vi "Dashboard Main.vi"() -> ()   [LabVIEW 2016]
uses:
  <vilib>/Utility/miscctls.llb/LVRowAndColumnTypeDef.ctl
  <vilib>/event_ctls.llb/eventvkey.ctl
  <vilib>/Rock Robotics/Network Tables/NT Read Numeric Array.vi
  <vilib>/Rock Robotics/WPI/Dashboard/WPI_DashboardLogging Global.vi
panel:
  in  "rect":T1
  in  "Camera Settings Right":T2={"Frame Rate"=30, "Compression"=30, "Size"=1, "DB Camera Config"=FALSE} {"Frame Rate" scale=1.0..30.0; "Compression" scale=100.0..-1.0; "Size" items=["640x480", "320x240", "160x120"]}
  in  "Camera Name Right":string(combo)="No Camera Selection"
  out "Camera Info":cluster{"Mbps LED":bool, "Mbps":dbl, "fps":dbl} {"fps" format="%#.1g"; "Mbps" format="%#.1g"}
  in  "Camera Settings":T2={"Frame Rate"=30, "Compression"=30, "Size"=1, "DB Camera Config"=FALSE} {"Frame Rate" scale=1.0..30.0; "Compression" scale=100.0..-1.0; "Size" items=["640x480", "320x240", "160x120"]}
  in  "TCP":refnum<k5>
  in  "Rec Mode":enum32{"Stop", "Record", "Playback"}(radio)
  out "Robot IP":string
  out "Image Message":string="Timeout in Camera Communications"
  in  "Dashboard Tab":T3(tab)
  in  "Select Auto":string(combo)="Select Autonomous ..."
  out "NT Connection":bool
  out "MotorChart R":cluster{"Numeric":dbl, "Numeric":dbl}(graph)
  out "MotorChart L":cluster{"Numeric":dbl, "Numeric":dbl}(graph)
  out "MotorSliders R":cluster{"MotorSlide1":dbl, "MotorSlide2":dbl} {"MotorSlide2" scale=-1.0..1.0 scale format="%#_2e"; "MotorSlide1" scale=-1.0..1.0 scale format="%#_2e"}
  out "MotorSliders L":cluster{"MotorSlide1":dbl, "MotorSlide2":dbl} {"MotorSlide2" scale=-1.0..1.0 scale format="%#_2e"; "MotorSlide1" scale=-1.0..1.0 scale format="%#_2e"}
  out "Gyro":dbl(knob) scale=0.0..360.0
  out "JS1 Z":dbl(slide) scale=-1.0..1.0 scale format="%#_2e"
  out "JS1 Graph":cluster{"X":dbl, "Y":dbl}[](graph)
  out "JS1 Buttons":T4
  out "JS2 Z":dbl(slide) scale=-1.0..1.0 scale format="%#_2e"
  out "JS2 Graph":cluster{"X":dbl, "Y":dbl}[](graph)
  out "JS2 Buttons":T4
  out "Mode":T5(ring)=enum."Auto Disabled"
  out "Camera Image Right":T6(plugin-control)
  in  "DB/String 9":string
  in  "DB/String 8":string
  in  "DB/String 7":string
  in  "DB/String 6":string
  in  "DB/String 5":string
  in  "DB/String 4":string
  in  "DB/String 3":string
  in  "DB/String 2":string
  in  "DB/String 1":string
  in  "DB/String 0":string
  in  "DB/Slider 0":dbl(slide) scale=0.0..5.0
  in  "DB/Slider 1":dbl(slide) scale=0.0..5.0
  in  "DB/Slider 2":dbl(slide) scale=0.0..5.0
  in  "DB/Slider 3":dbl(slide) scale=0.0..5.0
  out "DB/LED 3":bool
  out "DB/LED 2":bool
  out "DB/LED 1":bool
  out "DB/LED 0":bool
  in  "DB/Button 3":bool
  in  "DB/Button 2":bool
  in  "DB/Button 1":bool
  in  "DB/Button 0":bool caption="New Name"
  in  "Test Slider":dbl(slide) scale=0.0..100.0 scale format="%#_3g"
  in  "On/Off":bool caption="Solenoid"
  in  "Test Name":u16(ring) items=["Select the test to run..."]
  in  "Test Tree":string(tree)
  in  "Motor":cluster{"Value":dbl, "Enable":bool} {"Value" scale=-1.0..1.0 scale format="%#_3g"}
  out "Progress":T7 {"Test Progress" scale=0.0..100.0}
  in  "Rev/Fwd":cluster{"Forward":bool, "Reverse":bool}
  in  "Test Ring":u16(ring) items=["Monochrome", "Color"]
  out "Cmd Status":string
  in  "Execute Command":bool
  in  "Command Params":string[][](table)
  in  "Command Selection":i32(listbox)
  in  "CheckList":i32(listbox)
  out "Tree":string(tree)
  out "Camera Image":T6(plugin-control)
  out "Background":bool
  in  "Camera Name":string(combo)="No Camera Selection"
  # "HW"
  # "HW"
  # "Joysticks"
  # "Drive Motors"
  # "Front"
  # "Right"
  # "Left"
  # "Back"
  # "This tab is a great place for autonomous settings and robot-specific values.\nPlace controls and indicators inside this tab and match name to\nDashboard Variables on robot. You can also delete this comment."
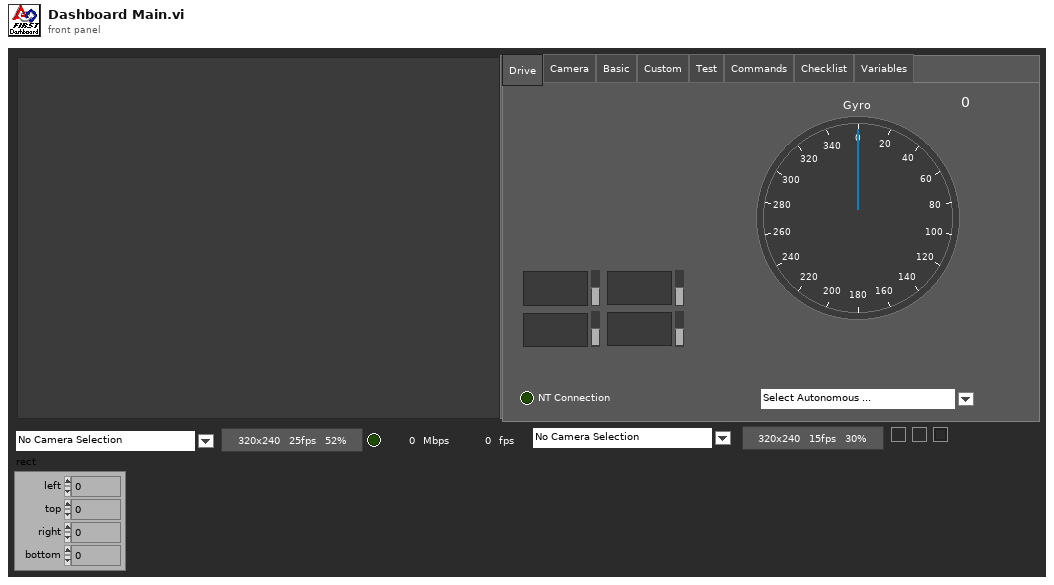
[diagram p1: front panel]
types:
  T1 = cluster{"left":i16, "top":i16, "right":i16, "bottom":i16}
  T2 = cluster{"Frame Rate":i32, "Compression":i32, "Size":u16, "DB Camera Config":bool}
  T3 = enum32{"Drive", "Camera", "Basic", "Custom", "Test", "Commands", "Checklist", "Variables"}
  T4 = cluster{bool, bool, bool, bool, bool, bool, bool, bool, bool, bool, bool, bool}
  T5 = enum8{"Tele-Op Disabled", "Tele-Op Enabled", "Auto Disabled", "Auto Enabled", "Test Disabled", "Test Enabled", "Disconnected", "No Code", "E-Stop"}
  T6 = typedef "IMAQ Image.ctl" = refnum<image>
  T7 = cluster{"Test Progress":u8, "Test Progress Text":string}
  T8 = typedef "Image Type" = u32
  T9 = cluster{"IDs":cluster{"RPC field ID":u16, "Unique ID":u16}, "String":string}
  T10 = enum32{"Drive", "Basic", "Custom", "Test", "Checklist", "Variables"}
  T11 = cluster{"Error Strings":string, "Disable Counts":cluster{u16, u16}, "Rail Faults":cluster{u16, u16, u16}, "Robot IP":string, "DB Mode":u8, "Event Info":cluster{"Name":string, "Type":u8, "Number":u16, "Replay":u8}}
  T12 = cluster{"Storage":cluster{"Disk Free":u64, "RAM Block":u32, "RAM free":u32}, "CPU Utilization":cluster{"CPU % ISR":sgl, "CPU % Time Crit":sgl, "CPU % Timed Str":sgl, "CPU % High":sgl, "CPU % Above":sgl, "CPU % Normal":sgl, "CPU % Low":sgl}, "CAN":cluster{"% Bus Utilization":sgl, "Bus Off Cnt":u32, "TX_FIFO Full Cnt":u32, "Receive Error Cnt":u8, "Transmit Error Cnt":u8}, "HID":cluster{"HID Outputs":u32, "Rumble Low":u16, "Rumble High":u16}[]}
  T13 = cluster{"Status bits":cluster{"Test Mode":bool, "Autonomous":bool, "Enabled":bool, "Code Start":bool, "Brownout":bool, "Reserved 2":bool, "Reserved 3":bool, "E-Stop":bool}, "Code Trace":cluster{"Disabled":bool, "TeleOp":bool, "Auto":bool, "Test":bool}, "Controller Type":enum16{"unknown", "cRIO", "roboRio"}, "Code?":enum16{"unknown", "noCode", "code"}, "Battery V":dbl}
  T14 = cluster{"Control Bits":cluster{"TestMode":bool, "Autonomous":bool, "Enabled":bool, "FMS Present":bool, bool, bool, bool, "E-Stop":bool}, "Team Station ":u8, "Countdown":sgl, "Joystick Values":cluster{"Axes":dbl[], "Buttons":bool[], "POVs":i16[]}[]}
  T15 = cluster{"Axes":dbl[], "Buttons":bool[], "POVs":i16[]}[]
  T16 = cluster{"Axes":dbl[], "Buttons":bool[], "POVs":i16[]}
  T17 = cluster{"Buttons[0]":bool, "Buttons[1]":bool, "Buttons[2]":bool, "Buttons[3]":bool, "Buttons[4]":bool, "Buttons[5]":bool, "Buttons[6]":bool, "Buttons[7]":bool, "Buttons[8]":bool, "Buttons[9]":bool, "Buttons[10]":bool, "Buttons[11]":bool}
  T18 = cluster{"Camera Image":refnum<vi>, "Dashboard Tab":refnum<vi>, "Background":refnum<vi>, "Rec Mode":refnum<vi>, "Test Slider":refnum<vi>, "On/Off ":refnum<vi>, "Test Ring":refnum<vi>, "Rev/Fwd":refnum<vi>, "Test Name":refnum<vi>, "Motor":refnum<vi>, "Progress":refnum<vi>, "CheckList":refnum<vi>, "Tree":refnum<vi>, "Test Tree":refnum<vi>, "Command Params":refnum<vi>, "Command Selection":refnum<vi>, "Execute Command":refnum<vi>, "Cmd Status":refnum<vi>, "Camera Settings":refnum<vi>, "Camera Name":refnum<vi>, "Camera Info":refnum<vi>, "Camera Settings Right":refnum<vi>, "Camera Name Right":refnum<vi>, "Camera Image Right":refnum<vi>}
  T19 = cluster{"Operation":enum16{"Update", "Clear"}, "Color Box":u32}[]
  T20 = typedef "eventvkey.ctl" = enum16{"ASCII", "Enter", "Return", "Shift", "Ctrl", "Alt", "Cmd", "Opt", "Caps", "NumLock", "Clear", "Break", "Up", "Down", "Left", "Right", "Insert", "Delete", "Home", "End", "PageUp", "PageDown", "Escape", "Help", "Pause", "ScrollLock", "F1", "F2", "F3", "F4", "F5", "F6", "F7", "F8", "F9", "F10", "F11", "F12", "F13", "F14", "F15", "F16", "F17", "F18", "F19", "F20", "F21", "F22", "F23", "F24", "Play", "VolumeUp", "VolumeDown", "Mute", "Two Byte Char"}
  T21 = cluster{"Image Size":bool, "Image Type":bool, "Pixel Value":bool, "ROI Information":bool, "Zoom Factor":bool}
  T22 = cluster{"Operation":enum16{"Update", "Clear"}, "Color Box":u32}
  T23 = typedef "LVRowAndColumnTypeDef.ctl" = cluster{"Row":i32, "Column":i32}
  T24 = cluster{"Shift":bool, "Ctrl":bool, "Alt":bool, "Cmd":bool, "Opt":bool}
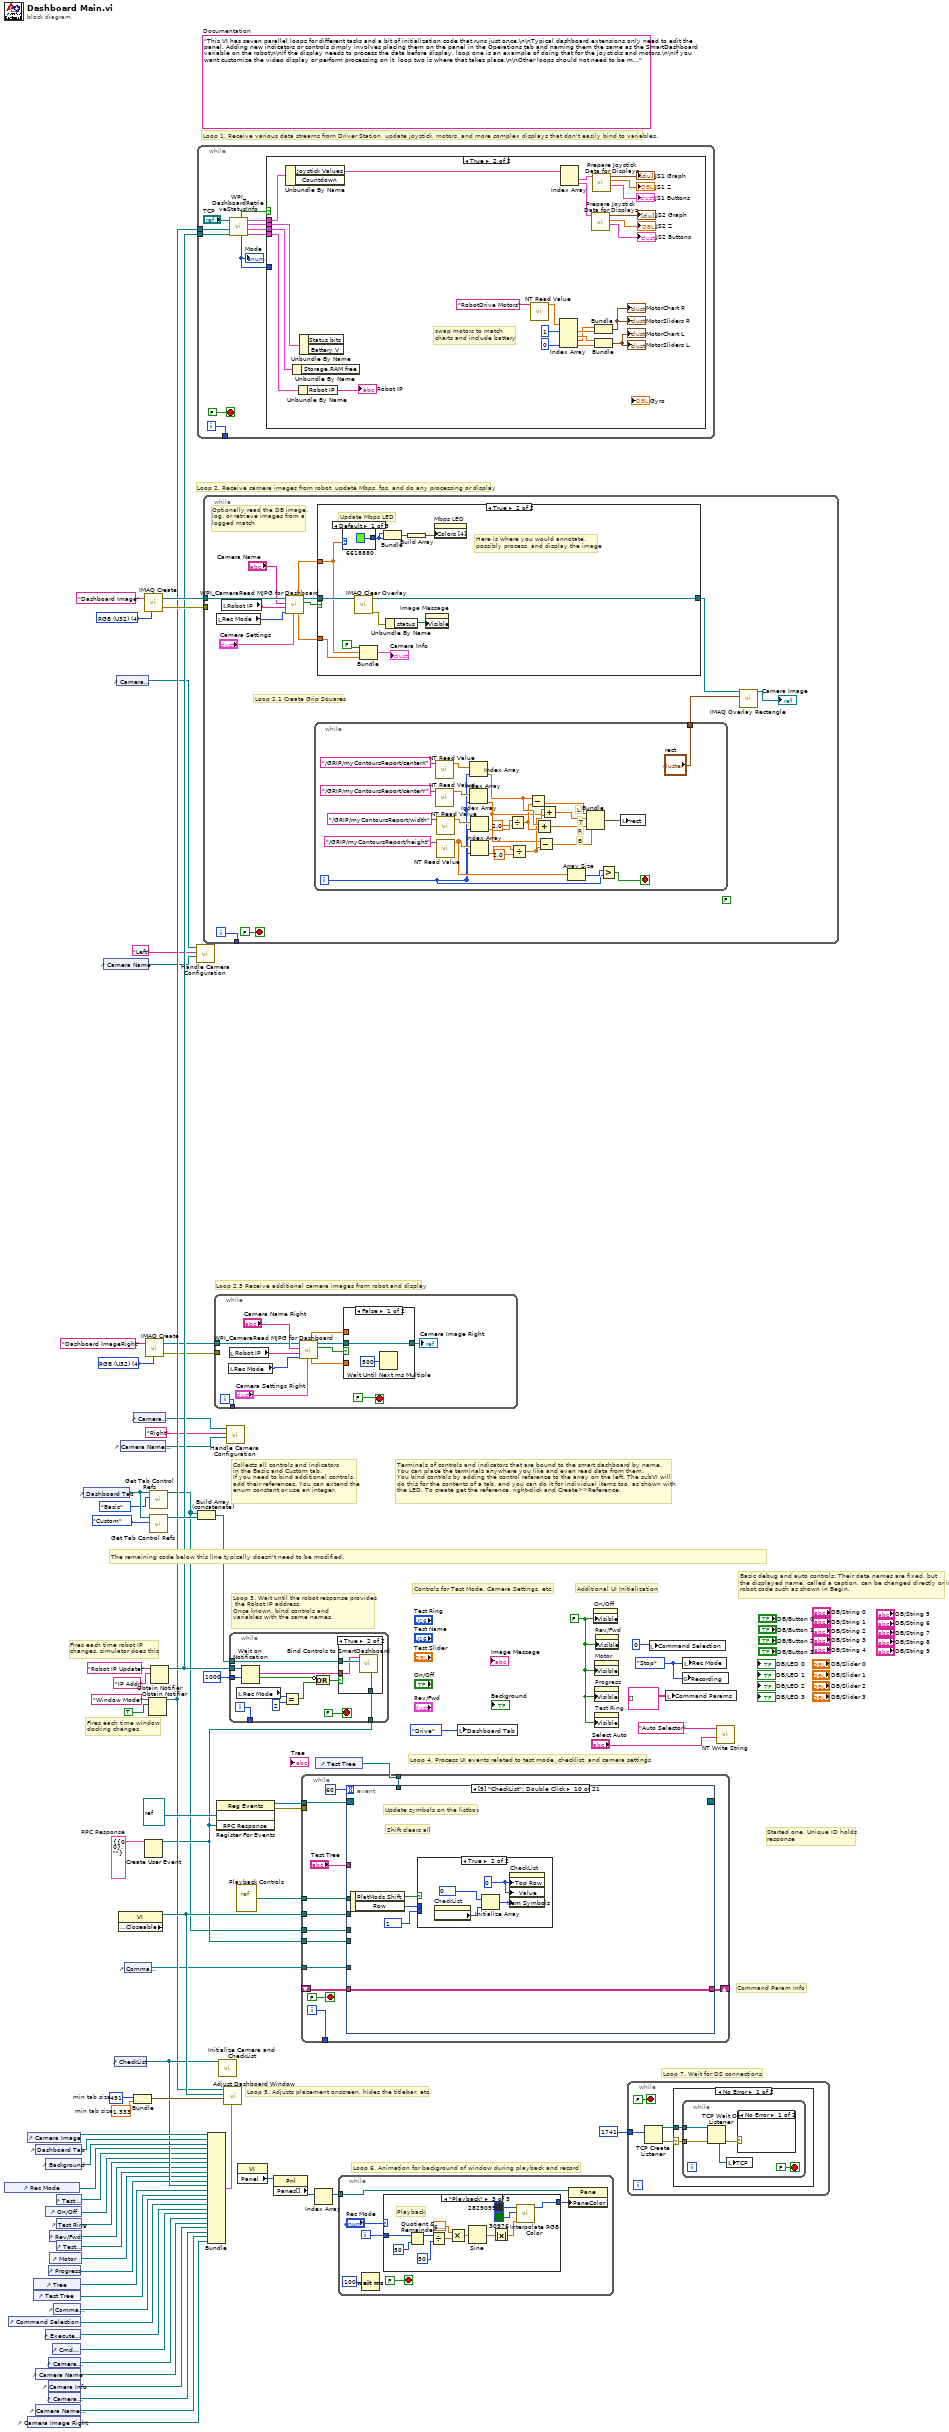
[diagram p0: block diagram]
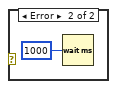
[diagram p3: hidden frame]
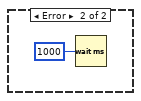
[diagram p4: hidden frame]
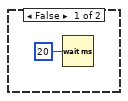
[diagram p5: hidden frame]
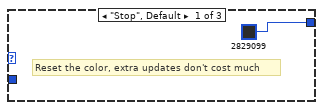
[diagram p6: hidden frame]
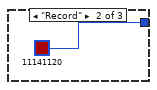
[diagram p7: hidden frame]
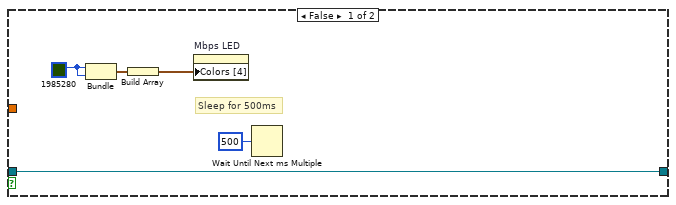
[diagram p9: hidden frame]
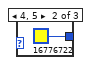
[diagram p10: hidden frame]
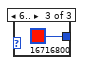
[diagram p11: hidden frame]
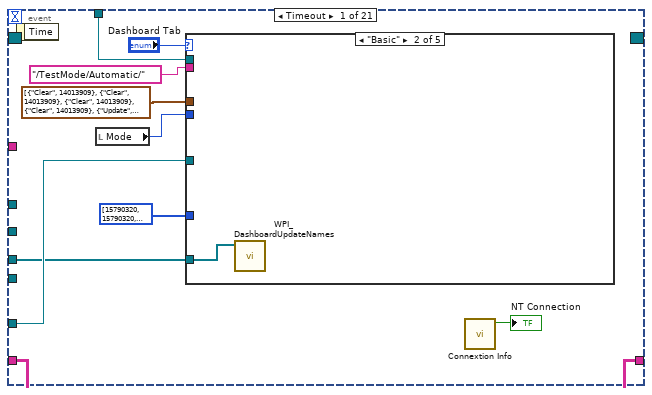
[diagram p12: hidden frame]
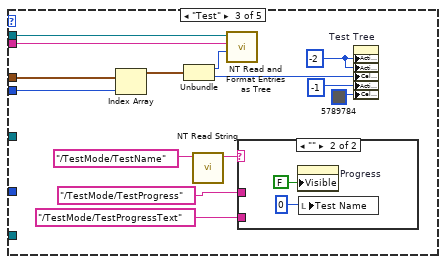
[diagram p14: hidden frame]
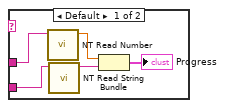
[diagram p15: hidden frame]
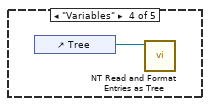
[diagram p16: hidden frame]
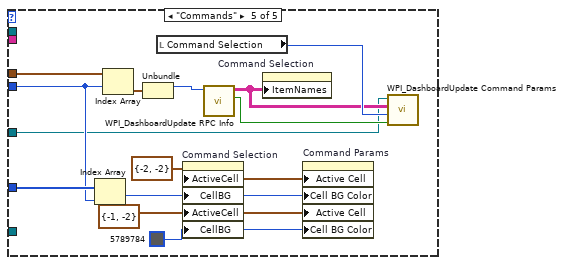
[diagram p17: hidden frame]
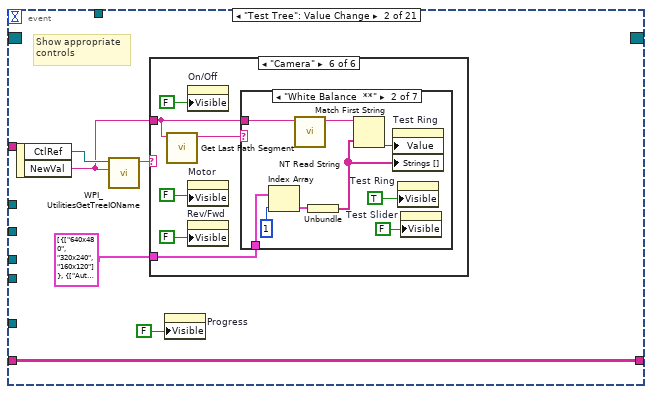
[diagram p18: hidden frame]
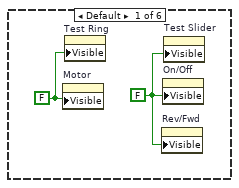
[diagram p19: hidden frame]
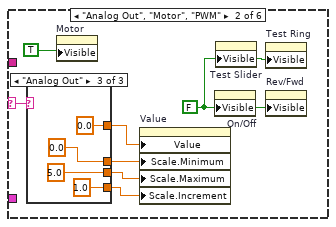
[diagram p20: hidden frame]
diagram:
  w10 = T8 4 items=["Grayscale (U8)", "Grayscale (I16)", "Grayscale (SGL)", "Complex (CSG)", "RGB (U32)", "HSL (U32)", "RGB (U64)"] ("Image Type")
  w26 = T9 {"IDs"={"RPC field ID"=0, "Unique ID"=0}, "String"=""}  # RPC Response
  w51 = 491  # min tab size
  w50 = 1.333  # min tab size
  w58 = enum32{"Stop", "Record", "Playback"}."Stop" ("Rec Mode")
  w33 = FALSE ("Visible")
  (unwired) "This VI has seven parallel loops for different tasks and a bit of initialization code that runs just once.\n\nTypical dashboard extensions only need to edit the panel. Adding new indicators or controls simply involves placing them on the panel in the Operations tab and naming them the same as the SmartDashboard variable on the robot\n\nIf the display needs to process the data before display, loop one is an example of doing that for the joysticks and motors.\n\nIf you want customize the video display or perform processing on it, loop two is where that takes place.\n\nOther loops should not need to be modified. They are pretty standard, and document the task they perform."  # Documentation
  w75 = T8 4 items=["Grayscale (U8)", "Grayscale (I16)", "Grayscale (SGL)", "Complex (CSG)", "RGB (U32)", "HSL (U32)", "RGB (U64)"] ("Image Type")
  # "Loop 2.5 Receive additional camera images from robot and display"
  # "Command Param Info"
  # "Started one, Unique ID holds\nresponse"
  # "Loop 7. Wait for DS connections"
  # "Basic debug and auto controls: Their data names are fixed, but\nthe displayed name, called a caption, can be changed directly or in\nrobot code such as shown in Begin."
  # "Controls for Test Mode, Camera Settings, etc."
  # "Additional UI Initialization"
  # "Loop 6. Animation for background of window during playback and record"
  # "Fires each time robot IP\nchanges, simulator does this"
  # "Fires each time window\ndocking changes."
  # "Collects all controls and indicators\nin the Basic and Custom tab.\nIf you need to bind additional controls,\nadd their references. You can extend the\nenum constant or use an integer."
  # "The remaining code below this line typically doesn't need to be modified."
  # "Loop 4. Process UI events related to test mode, checklist, and camera settings"
  # "Terminals of controls and indicators that are bound to the smart dashboard by name.\nYou can place the terminals anywhere you like and even read data from them.\nYou bind controls by adding the control reference to the array on the left. The subVI will\ndo this for the contents of a tab, and you can do it for individual items too, as shown with\nthe LED. To create get the reference, right-click and Create>>Reference."
  # "Loop 3. Wait until the robot response provides\n the Robot IP address.\nOnce known, bind controls and\nvariables with the same names."
  # "Loop 5. Adjusts placement onscreen, hides the titlebar, etc."
  # "Loop 1. Receive various data streams from Driver Station, update joystick, motors, and more complex displays that don't easily bind to variables."
  # "Loop 2. Receive camera images from robot, update Mbps, fps, and do any processing or display"
  n1 = control-ref of="Rec Mode"() -> (w39:refnum<vi>)
  n2 = control-ref of="Command Selection"() -> (w25:refnum<vi>)
  n3 = control-ref of="Camera Image Right"() -> (w1:refnum<vi>)
  n4 = control-ref of="Camera Image"() -> (w53:refnum<vi>)
  n5 = control-ref of="Tree"() -> (w43:refnum<vi>)
  n6 = control-ref of="Test Tree"() -> (w42:refnum<vi>)
  n7 = control-ref of="Dashboard Tab"() -> (w52:refnum<vi>)
  n8 = control-ref of="Camera Name"() -> (w16:refnum<vi>)
  n9 = control-ref of="Camera Name Right"() -> (w2:refnum<vi>)
  n10 = control-ref of="Execute Command"() -> (w27:refnum<vi>)
  n11 = control-ref of="Background"() -> (w48:refnum<vi>)
  n12 = control-ref of="On/Off"() -> (w37:refnum<vi>)
  n13 = control-ref of="Progress"() -> (w34:refnum<vi>)
  n14 = control-ref of="Camera Settings"() -> (w17:refnum<vi>)
  n15 = control-ref of="Camera Info"() -> (w15:refnum<vi>)
  n16 = control-ref of="Camera Settings Right"() -> (w3:refnum<vi>)
  n17 = control-ref of="Rev/Fwd"() -> (w35:refnum<vi>)
  n18 = control-ref of="Motor"() -> (w40:refnum<vi>)
  n19 = control-ref of="Cmd Status"() -> (w21:refnum<vi>)
  n20 = control-ref of="Command Params"() -> (w28:refnum<vi>)
  n21 = control-ref of="Test Slider"() -> (w38:refnum<vi>)
  n22 = control-ref of="Test Ring"() -> (w36:refnum<vi>)
  n23 = control-ref of="Test Name"() -> (w41:refnum<vi>)
  n24 = control-ref of="Dashboard Tab"() -> (w56:refnum<vi>)
  n25 = control-ref of="Camera Name"() -> (w18:refnum<vi>)
  n26 = control-ref of="CheckList"() -> (w44:refnum<vi>)
  n27 = control-ref of="Camera Settings"() -> (w19:refnum<vi>)
  n28 = property class="VI" props=["Front Panel.Closeable"]() -> (reference out=w57:refnum<vi>)  [unwired: 2 in, 2 out]
  n29 = control-ref of="Camera Name Right"() -> (w6:refnum<vi>)
  n30 = control-ref of="Command Params"() -> (w20:refnum<vi>)
  n31 = control-ref of="Camera Settings Right"() -> (w7:refnum<vi>)
  n32 = Bundle("min tab size"=w51, "min tab size"=w50) -> (w49:cluster{"min tab size":i32, "min tab size":dbl})  [unwired: 1 in]
  n33 = call "IMAQ Create"("Image Name"="Dashboard Image", "Image Type"=w75) -> ("New Image"=w73:T6, "error out"=w72:errorcluster)  [unwired: 2 in, 1 out]
  n34 = Create User Event(user event datatype=w26) -> (user event=w22:refnum<user-event>)  [unwired: 1 in, 1 out]
  n35 = call "IMAQ Create"("Image Name"="Dashboard ImageRight", "Image Type"=w10) -> ("New Image"=w9:T6, "error out"=w8:errorcluster)  [unwired: 2 in, 1 out]
  n36 = Obtain Notifier(name (unnamed)="Window Mode", notification data type=TRUE) -> (notifier out=w31:refnum<notifier>)  [unwired: 2 in, 2 out]
  n37 = call <vilib>:"Get Tab Control Refs.vi"("Page Index"=T10."Basic" ("Dashboard Tab"), "TabControl in"=w56) -> ("ControlsOnPage"=w14:refnum<vi>[])  [unwired: 9 in]
  n38 = call <vilib>:"Get Tab Control Refs.vi"("Page Index"=T10."Custom" ("Dashboard Tab"), "TabControl in"=w56) -> ("ControlsOnPage"=w55:refnum<vi>[])  [unwired: 9 in]
  n39 = Obtain Notifier(name (unnamed)="Robot IP Update", notification data type="IP Addr" ("name (unnamed)")) -> (notifier out=w32:refnum<notifier>)  [unwired: 2 in, 2 out]
  n40 = call "Handle Camera Configuration.vi"("CameraNameRef"=w18, "Camera File Name"="Left", "ClusterRef"=w19) -> ()  [unwired: 9 in]
  n41 = Build Array (concatenate)(w14, w55) -> (w54:refnum<vi>[])
  n42 = while {
    tunnel: [w85] -> _
    tunnel: w32 -> [w79]
    tunnel: w31 -> [w76]
    i -> [w85]
    stop <- FALSE stop-if-true
    n43 = call <vilib>:"WPI_DashboardRetrieveStatusInfo.vi"("Binding Refnum"=w79, "Window Mode Notifier"=w76, "TCP Cnx"="TCP") -> ("Power and Errors"=w80:T11, "Robot Metrics"=w83:T12, "Status Info"=w84:T13, "Control Info"=w81:T14, "Robot Mode"=w78:T5, "Process?"=w82:bool)  [unwired: 3 in]
    "Mode" <- w78
    n44 = case shown="True" w82 {
      tunnel: w84 -> [_ w111]
      tunnel: w83 -> [_ w110]
      tunnel: w81 -> [_ w109]
      tunnel: w80 -> [_ w108]
      tunnel: w78 -> [_ _]
      frame False {
        n45 = Wait (ms)(milliseconds to wait=u32 20) -> ()  [unwired: 1 out]
      }
      frame True {
        # "swap motors to match\ncharts and include battery"
        n46 = Unbundle By Name(w109) -> ("Joystick Values"=w99:T15)  [unwired: 1 out]
        n47 = Unbundle By Name(w110) -> ()  [unwired: 1 out]
        n48 = Unbundle By Name(w108) -> ("Robot IP"=→"Robot IP":string)
        n49 = Unbundle By Name(w111) -> ()  [unwired: 2 out]
        n50 = call-poly <vilib>:"NT Read Value.vi"("Name"="RobotDrive Motors") -> ("Numeric Array"=w89:dbl[])  [unwired: 9 in, 1 out]
        n51 = Index Array(array=w89, index #1=1, index #4=0) -> (element #1=w103:dbl, element #2=w104:dbl, element #3=w102:dbl, element #4=w107:dbl)  [unwired: 2 in]
        n52 = Index Array(array=w99) -> (element #1=w98:T16, element #2=w94:T16)  [unwired: 2 in]
        n53 = call "Prepare Joystick Data for Displays.vi"("Joystick Values"=w94) -> ("Buttons"=→"JS2 Buttons":T17, "Z Axis"=→"JS2 Z":dbl, "Cartesian Data"=→"JS2 Graph":cluster{"X axis":dbl, "X axis":dbl}[])  [unwired: 8 in]
        n54 = call "Prepare Joystick Data for Displays.vi"("Joystick Values"=w98) -> ("Buttons"=→"JS1 Buttons":T17, "Z Axis"=→"JS1 Z":dbl, "Cartesian Data"=→"JS1 Graph":cluster{"X axis":dbl, "X axis":dbl}[])  [unwired: 8 in]
        n55 = Bundle("Numeric"=w102, "Numeric"=w103) -> (→"MotorChart R" →"MotorSliders R":cluster{"Numeric":dbl, "Numeric":dbl})  [unwired: 1 in]
        n56 = Bundle("Numeric"=w104, "Numeric"=w107) -> (→"MotorChart L" →"MotorSliders L":cluster{"Numeric":dbl, "Numeric":dbl})  [unwired: 1 in]
      }
    }
  }
  n57 = while {
    tunnel: w73 -> [w123]
    tunnel: w72 -> [_]
    tunnel: [w124] -> _
    i -> [w124]
    stop <- FALSE stop-if-true
    (unwired) FALSE
    # "Loop 2.1 Create Grip Squares"
    # "Optionally read the DB image,\nlog, or retrieve images from a\nlogged match"
    n58 = local read "Rec Mode"() -> (w119:enum32{"Stop", "Record", "Playback"})
    n59 = local read "Robot IP"() -> (w118:string)
    n60 = call <vilib>:"WPI_CameraRead MJPG for Dashboard.vi"("Camera Settings"="Camera Settings", "Rec Mode"=w119, "Robot IP"=w118, "Camera Name"="Camera Name", "Refnum in"=w123) -> ("Active"=w121:bool, "Refnum out"=w122:T6, "FPS"=w120:dbl, "Bandwidth (Mbps)"=w117:dbl)  [unwired: 3 in]
    n61 = while {
      tunnel: ["rect"] -> w114
      i -> [w139]
      stop <- w144 stop-if-true
      # "B"
      # "R"
      # "T"
      # "L"
      n62 = call-poly <vilib>:"NT Read Value.vi"("Name"="/GRIP/myContoursReport/centerX") -> ("Numeric Array"=w143:dbl[])  [unwired: 9 in, 1 out]
      n63 = call-poly <vilib>:"NT Read Value.vi"("Name"="/GRIP/myContoursReport/centerY") -> ("Numeric Array"=w142:dbl[])  [unwired: 9 in, 1 out]
      n64 = call-poly <vilib>:"NT Read Value.vi"("Name"="/GRIP/myContoursReport/height") -> ("Numeric Array"=w140:dbl[])  [unwired: 9 in, 1 out]
      n65 = call-poly <vilib>:"NT Read Value.vi"("Name"="/GRIP/myContoursReport/width") -> ("Numeric Array"=w141:dbl[])  [unwired: 9 in, 1 out]
      n66 = Index Array(array=w143, index=w139) -> (element=w135:dbl)
      n67 = Index Array(array=w142, index=w139) -> (element=w129:dbl)
      n68 = Index Array(array=w141, index=w139) -> (element=w138:dbl)
      n69 = Index Array(array=w140, index=w139) -> (element=w131:dbl)
      n70 = Divide(x=w138, y=2.0) -> (x/y=w134:dbl)
      n71 = Divide(x=w131, y=2.0) -> (x/y=w130:dbl)
      n72 = Subtract(x=w135, y=w134) -> (x-y=w136:dbl)
      n73 = Add(x=w135, y=w134) -> (x+y=w133:dbl)
      n74 = Subtract(x=w129, y=w130) -> (x-y=w128:dbl)
      n75 = Add(x=w129, y=w130) -> (x+y=w127:dbl)
      n76 = Array Size(array=w140) -> (size(s)=w145:i32)
      n77 = Bundle(w136, w127, w133, w128) -> (w146:cluster{dbl, dbl, dbl, dbl})  [unwired: 1 in]
      n78 = Greater?(x=w145, y=w139) -> (0:w144:bool)
      n79 = local write "rect"(w146) -> ()
    }
    n80 = case shown="True" w121 {
      tunnel: w122 -> [w151 w162]
      tunnel: w117 -> [_ w159]
      tunnel: w120 -> [_ w160]
      tunnel: [w151 w156] -> w113
      frame False {
        w153 = u32 1985280 ("Color Box")
        # "Sleep for 500ms"
        n81 = Bundle("Color Box"=w153, "Color Box"=w153) -> (w154:cluster{"Color Box":u32, "Color Box":u32})  [unwired: 1 out]
        n82 = Build Array(w154) -> (w152:cluster{"Color Box":u32, "Color Box":u32}[])
        n83 = property on="Mbps LED" class="Bool (strict)"("Colors [4]"=w152) -> ()  [unwired: 2 in, 2 out]
        n84 = Wait Until Next ms Multiple(millisecond multiple=u32 500) -> ()  [unwired: 1 out]
      }
      frame True {
        # "Here is where you would annotate,\npossibly process, and display the image"
        # "Update Mbps LED"
        n85 = case shown="Default" w159 {
          tunnel: [u32 6618880 ("Color Box") u32 16776722 ("Color Box") u32 16716800 ("Color Box")] -> w163
          frame Default {
          }
          frame 4, 5 {
          }
          frame 6.. {
          }
        }
        n86 = call "IMAQ Clear Overlay"("Image"=w162) -> ("error out"=w165:errorcluster, "Image Out"=w156:T6)  [unwired: 2 in, 7 out]
        n87 = Bundle(FALSE, "Bandwidth (Mbps)"=w159, "FPS"=w160) -> (→"Camera Info":cluster{bool, "Bandwidth (Mbps)":dbl, "FPS":dbl})  [unwired: 1 in]
        n88 = Bundle("Color Box"=w163, "Color Box"=w163) -> (w164:cluster{"Color Box":u32, "Color Box":u32})  [unwired: 1 out]
        n89 = Unbundle By Name(w165) -> ("status"=w166:bool)
        n90 = Build Array(w164) -> (w161:cluster{"Color Box":u32, "Color Box":u32}[])
        n91 = property on="Image Message" class="Str"("Visible"=w166) -> ()  [unwired: 2 in, 2 out]
        n92 = property on="Mbps LED" class="Bool (strict)"("Colors [4]"=w161) -> ()  [unwired: 2 in, 2 out]
      }
    }
    n93 = call "IMAQ Overlay Rectangle"("Rectangle"=w114, "Image"=w113) -> ("Image Out"=→"Camera Image":T6)  [unwired: 8 in, 1 out]
  }
  n94 = Bundle("Camera Image"=w53, "Dashboard Tab"=w52, "Background"=w48, "Rec Mode"=w39, "Test Slider"=w38, "On/Off"=w37, "Test Ring"=w36, "Rev/Fwd"=w35, "Test Name"=w41, "Motor"=w40, "Progress"=w34, "CheckList"=w44, "Tree"=w43, "Test Tree"=w42, "Command Params"=w28, "Command Selection"=w25, "Execute Command"=w27, "Cmd Status"=w21, "Camera Settings"=w17, "Camera Name"=w16, "Camera Info"=w15, "Camera Settings Right"=w3, "Camera Name Right"=w2, "Camera Image Right"=w1) -> (w45:T18)  [unwired: 1 in]
  n95 = while {
    tunnel: w9 -> [w180]
    tunnel: w8 -> [_]
    tunnel: [w174] -> _
    i -> [w174]
    stop <- FALSE stop-if-true
    n96 = local read "Rec Mode"() -> (w178:enum32{"Stop", "Record", "Playback"})
    n97 = local read "Robot IP"() -> (w179:string)
    n98 = call <vilib>:"WPI_CameraRead MJPG for Dashboard.vi"("Camera Settings"="Camera Settings Right", "Rec Mode"=w178, "Robot IP"=w179, "Camera Name"="Camera Name Right", "Refnum in"=w180) -> ("Active"=w173:bool, "Refnum out"=w176:T6, "FPS"=w171:dbl, "Bandwidth (Mbps)"=w172:dbl)  [unwired: 3 in]
    n99 = case shown="False" w173 {
      tunnel: w176 -> [w182 w184]
      tunnel: w172 -> [_ _]
      tunnel: w171 -> [_ _]
      tunnel: [w182 w184] -> w170
      frame False {
        n100 = Wait Until Next ms Multiple(millisecond multiple=u32 500) -> ()  [unwired: 1 out]
      }
      frame True {
      }
    }
    "Camera Image Right" <- w170
  }
  n101 = register-events(refnum<vi> refnum, w22) -> (reference out=w62:refnum<event-registration>, error out=w61:errorcluster)  [unwired: 2 in]
  n102 = call "Initialize Camera and CheckList.vi"("ListBox in"=w44) -> ()  [unwired: 11 in]
  n103 = call "Adjust Dashboard Window.vi"("Sizing Refnums"=w45, "Size Constraints"=w49, "VI"=w57, "WIn Mode"=w31) -> ()  [unwired: 8 in]
  n104 = call "Handle Camera Configuration.vi"("CameraNameRef"=w6, "Camera File Name"="Right", "ClusterRef"=w7) -> ()  [unwired: 9 in]
  n105 = while {
    tunnel: w54 -> [w196]
    tunnel: w32 -> [w194]
    tunnel: [w192] -> _
    tunnel: u32 1000 ("milliseconds to wait") -> [w191]
    tunnel: w22 -> [w185]
    i -> [w192]
    stop <- FALSE stop-if-true
    n106 = local read "Rec Mode"() -> (w187:enum32{"Stop", "Record", "Playback"})
    n107 = Wait on Notification(notifier=w194, timeout in ms (-1)=w191) -> (notification=w193:string, timed out?=w189:bool)  [unwired: 2 in, 2 out]
    n108 = Equal?(x=w187, y=u16 2 ("Rec Mode")) -> (x = y?=w188:bool)
    n109 = Compound Arithmetic op=OR(invert w189, w188) -> (w190:bool)
    n110 = case shown="True" w190 {
      tunnel: w196 -> [_ w199]
      tunnel: w193 -> [_ w198]
      tunnel: w185 -> [_ w197]
      frame False {
      }
      frame True {
        n111 = call <vilib>:"Bind Controls to SmartDashboard.vi"("RPC ref"=w197, "Bound Control Refs"=w199, "Server IP Address"=w198) -> ()  [unwired: 9 in]
      }
    }
  }
  n112 = vi-ref "Playback Controls.vi"() -> (w63:refnum<vi>)
  n113 = property class="VI"() -> ("Panel"=w65:refnum<vi>)  [unwired: 2 in, 2 out]
  n114 = property class="Pnl"(reference=w65) -> ("Panes[]"=w66:refnum<vi>[])  [unwired: 1 in, 2 out]
  n115 = Index Array(array=w66) -> (element=w64:refnum<vi>)  [unwired: 1 in]
  n116 = control-ref of="Test Tree"() -> (w67:refnum<vi>)
  n117 = while {
    tunnel: [w209] -> _
    tunnel: w67 -> [w208]
    tunnel: w63 -> [w207]
    tunnel: w62 -> [w206]
    tunnel: w61 -> [_]
    tunnel: w57 -> [w205]
    tunnel: w22 -> [w204]
    tunnel: w20 -> [w203]
    shift-right: [w202] -> _
    shift-left: _ -> [w201]
    tunnel: w14 -> [w200]
    i -> [w209]
    stop <- FALSE stop-if-true
    n118 = event shown="[9] \"CheckList\": Double Click" {
      selector: w206 -> [_ _ _ _ _ _ _ _ _ _ _ _ _ _ _ _ _ _ _ _ _]
      dyn-events: [_ _ _ _ _ _ _ _ _ _ _ _ _ _ _ _ w465 _ _ _ _] -> _
      timeout: u32 60 ("milliseconds to wait") -> [_ _ _ _ _ _ _ _ _ _ _ _ _ _ _ _ _ _ _ _ _]
      tunnel: w208 -> [w221 _ _ _ _ _ _ _ _ _ _ _ _ _ _ _ _ _ _ _ _]
      tunnel: "Test Tree" -> [_ _ _ _ _ _ _ _ _ _ _ w432 w440 w442 w446 w454 _ _ _ _ _]
      tunnel: w207 -> [_ _ _ _ _ _ _ _ _ _ _ _ _ _ _ _ w467 _ w485 _ _]
      tunnel: w205 -> [_ _ _ _ _ _ _ _ _ _ _ _ _ _ _ _ w463 _ _ _ _]
      tunnel: w204 -> [_ _ _ _ _ _ _ _ _ _ _ _ _ _ _ _ w459 _ _ _ _]
      tunnel: w203 -> [w216 _ _ _ _ _ w383 _ _ _ _ _ _ _ _ _ _ _ _ _ _]
      tunnel: [w215 w260 w362 w367 w376 w380 w381 w390 w400 w407 w419 w431 w438 w441 w445 w453 w458 w480 w482 w486 w497] -> w202
      tunnel: w201 -> [w215 w260 w362 w367 w376 w380 w381 _ _ w407 w419 w431 w438 w441 w445 w453 w458 w480 w482 w486 w497]
      tunnel: w200 -> [w213 _ _ _ _ _ _ _ _ _ _ _ _ _ _ _ _ _ _ _ _]
      event Timeout {
        n119 = event-data() -> ()  [unwired: 1 in, 1 out]
        n120 = local read "Mode"() -> (w218:T5)
        n121 = case shown="\"Basic\"" "Dashboard Tab" {
          tunnel: w221 -> [_ _ w237 _ _]
          tunnel: "/TestMode/Automatic/" ("Name Pattern") -> [_ _ w236 _ _]
          tunnel: T19 [{"Operation"=enum."Clear", "Color Box"=14013909}, {"Operation"=enum."Clear", "Color Box"=14013909}, {"Operation"=enum."Clear", "Color Box"=14013909}, {"Operation"=enum."Clear", "Color Box"=14013909}, {"Operation"=enum."Update", "Color Box"=14013909}, {"Operation"=enum."Update", "Color Box"=16777215}, {"Operation"=enum."Clear", "Color Box"=14013909}, {"Operation"=enum."Clear", "Color Box"=14013909}, {"Operation"=enum."Clear", "Color Box"=14013909}] -> [_ _ w229 _ w253]
          tunnel: w218 -> [_ _ w228 _ w252]
          tunnel: u32[] [15790320, 15790320, 15790320, 15790320, 16777215, 16777215, 15790320, 15790320, 15790320] -> [_ _ _ _ w258]
          tunnel: w216 -> [_ _ _ _ w246]
          tunnel: w213 -> [_ w223 _ _ _]
          frame "Custom", Default {
          }
          frame "Basic" {
            n122 = call <vilib>:"WPI_DashboardUpdateNames.vi"("Controls on Tab"=w223) -> ()  [unwired: 11 in]
          }
          frame "Test" {
            w235 = -2 ("Active Item:Row Number")
            n123 = Index Array(array=w229, index=w228) -> (element=w230:T22)
            n124 = Unbundle(w230) -> ("Operation"=w231:enum16{"Update", "Clear"}, "Color Box"=w232:u32)
            n125 = call <vilib>:"NT Read String.vi"("Name"="/TestMode/TestName") -> ("String"=w226:string)  [unwired: 9 in, 1 out]
            n126 = call <vilib>:"NT Read and Format Entries as Tree.vi"("Operation"=w231, "Name Pattern"=w236, "Tree Refnum"=w237) -> ()  [unwired: 7 in, 2 out]
            n127 = case shown="\"\"" w226 {
              tunnel: "/TestMode/TestProgress" ("Name") -> [w239 _]
              tunnel: "/TestMode/TestProgressText" ("Name") -> [w238 _]
              frame Default {
                n128 = call <vilib>:"NT Read Number.vi"("Name"=w239) -> ("Numeric"=w240:dbl)  [unwired: 9 in, 1 out]
                n129 = call <vilib>:"NT Read String.vi"("Name"=w238) -> ("String"=w241:string)  [unwired: 9 in, 1 out]
                n130 = Bundle("Numeric"=w240, "String"=w241) -> (→"Progress":cluster{"Numeric":dbl, "String":string})  [unwired: 1 in]
              }
              frame "" {
                n131 = property on="Progress" class="Clust (strict)"("Visible"=FALSE) -> ()  [unwired: 2 in, 2 out]
                n132 = local write "Test Name"(u16 0) -> ()
              }
            }
            n133 = property on="Test Tree" class="Tree (strict)"("Active Item Row Number"=w235, "ActiveColNum"=w235, "CellBG"=w232, "Active Item Row Number"=-1 ("Active Item:Row Number"), "CellBG"=u32 5789784 ("Color Box")) -> ()  [unwired: 2 in, 2 out]
          }
          frame "Variables" {
            n134 = control-ref of="Tree"() -> (w245:refnum<vi>)
            n135 = call <vilib>:"NT Read and Format Entries as Tree.vi"("Tree Refnum"=w245) -> ()  [unwired: 9 in, 2 out]
          }
          frame "Commands" {
            w254 = u32 5789784 ("Color Box")
            w255 = T23 {"Row"=-1, "Column"=-2} ("Active Cell:Active Cell")
            w257 = T23 {"Row"=-2, "Column"=-2} ("Active Cell:Active Cell")
            n136 = Index Array(array=w258, index=w252) -> (element=w256:u32)
            n137 = Index Array(array=w253, index=w252) -> (element=w251:T22)
            n138 = Unbundle(w251) -> ("Operation"=w250:enum16{"Update", "Clear"})  [unwired: 1 out]
            n139 = local read "Command Selection"() -> (w249:i32)
            n140 = property on="Command Selection" class="MCListbox (strict)"("ActiveCell"=w257, "CellBG"=w256, "ActiveCell"=w255, "CellBG"=w254) -> ()  [unwired: 2 in, 2 out]
            n141 = call <vilib>:"WPI_DashboardUpdate RPC Info.vi"("Operation"=w250) -> ("update"=w248:bool, "commands"=w247:string[][])  [unwired: 9 in]
            n142 = property on="Command Selection" class="MCListbox (strict)"("ItemNames"=w247) -> ()  [unwired: 2 in, 2 out]
            n143 = property on="Command Params" class="Tbl (strict)"("Active Cell"=w257, "Cell BG Color"=w256, "Active Cell"=w255, "Cell BG Color"=w254) -> ()  [unwired: 2 in, 2 out]
            n144 = call <vilib>:"WPI_DashboardUpdate Command Params.vi"("Update"=w248, "NewVal"=w249, "Commands"=w247, "Param Tbl"=w246) -> ()  [unwired: 7 in, 1 out]
          }
        }
        n145 = call <vilib>:"Connextion Info.vi"() -> ("Connected"=→"NT Connection":bool)  [unwired: 10 in, 1 out]
      }
      event "Test Tree": Value Change {
        # "Show appropriate\ncontrols"
        n146 = event-data() -> ("CtlRef"=w263:refnum<vi>, "NewVal"=w261:string)  [unwired: 1 in]
        n147 = call <vilib>:"WPI_UtilitiesGetTreeIOName.vi"("NewVal"=w261, "TreeControl in"=w263) -> ("I/O Name"=w264:string)  [unwired: 9 in]
        n148 = case shown="\"Camera\"" w264 {
          selector: w264 -> [_ w271 _ w293 w302 _]
          tunnel: w261 -> [_ _ w290 w292 _ w309]
          tunnel: cluster{string[]}[] [{["640x480", "320x240", "160x120"]}, {["Auto", "Fixed indoor", "Fixed outdoor 1", "Fixed outdoor 2", "Fixed fluorescent 1", "Fixed fluorescent 2", "Hold current"]}, {["Auto", "Flicker-free 50 Hz", "Flicker-free 60 Hz", "Hold current"]}, {["None", "Prioritize frame rate", "Prioritize image quality"]}, {["Monochrome", "Color"]}] -> [_ _ _ _ _ w308]
          frame Default {
            w266 = FALSE ("Visible")
            w265 = FALSE ("Visible")
            n149 = property on="Motor" class="Clust (strict)"("Visible"=w265) -> ()  [unwired: 2 in, 2 out]
            n150 = property on="Test Ring" class="Ring (strict)"("Visible"=w265) -> ()  [unwired: 2 in, 2 out]
            n151 = property on="Rev/Fwd" class="Clust (strict)"("Visible"=w266) -> ()  [unwired: 2 in, 2 out]
            n152 = property on="On/Off" class="Bool (strict)"("Visible"=w266) -> ()  [unwired: 2 in, 2 out]
            n153 = property on="Test Slider" class="Slide (strict)"("Visible"=w266) -> ()  [unwired: 2 in, 2 out]
          }
          frame "Analog Out", "Motor", "PWM" {
            w272 = FALSE ("Visible")
            n154 = case shown="\"Analog Out\"" w271 {
              tunnel: [1.0 ("Value") -1.0 ("Value") 0.0 ("Value")] -> w270
              tunnel: [255.0 ("Value") 1.0 ("Value") 5.0 ("Value")] -> w269
              tunnel: [128.0 ("Value") 0.0 ("Value") 0.0 ("Value")] -> w268
              tunnel: [64.0 ("Value") 0.5 ("Value") 1.0 ("Value")] -> w267
              frame "PWM" {
              }
              frame "Motor", Default {
              }
              frame "Analog Out" {
              }
            }
            n155 = property on="Motor" class="Clust (strict)"("Visible"=TRUE) -> ()  [unwired: 2 in, 2 out]
            n156 = property on="Value" class="Slide (strict)"("Value"=w268, "Scale.Minimum"=w270, "Scale.Maximum"=w269, "Scale.Increment"=w267) -> ()  [unwired: 2 in, 2 out]
            n157 = property on="On/Off" class="Bool (strict)"("Visible"=w272) -> ()  [unwired: 2 in, 2 out]
            n158 = property on="Test Slider" class="Slide (strict)"("Visible"=w272) -> ()  [unwired: 2 in, 2 out]
            n159 = property on="Test Ring" class="Ring (strict)"("Visible"=w272) -> ()  [unwired: 2 in, 2 out]
            n160 = property on="Rev/Fwd" class="Clust (strict)"("Visible"=w272) -> ()  [unwired: 2 in, 2 out]
          }
          frame "Servo" {
            w288 = FALSE ("Visible")
            n161 = call <vilib>:"NT Read Number.vi"("Name"=w290) -> ("Numeric"=w289:dbl)  [unwired: 9 in, 1 out]
            n162 = property on="Test Slider" class="Slide (strict)"("Visible"=TRUE, "Scale.Maximum"=170.0 ("Scale.Range:Maximum")) -> ()  [unwired: 2 in, 2 out]
            n163 = local write "Test Slider"(w289) -> ()
            n164 = property on="Motor" class="Clust (strict)"("Visible"=w288) -> ()  [unwired: 2 in, 2 out]
            n165 = property on="Rev/Fwd" class="Clust (strict)"("Visible"=w288) -> ()  [unwired: 2 in, 2 out]
            n166 = property on="On/Off" class="Bool (strict)"("Visible"=w288) -> ()  [unwired: 2 in, 2 out]
            n167 = property on="Test Ring" class="Ring (strict)"("Visible"=w288) -> ()  [unwired: 2 in, 2 out]
          }
          frame "Relay", "Solenoid" {
            w291 = FALSE ("Visible")
            n168 = property on="Motor" class="Clust (strict)"("Visible"=w291) -> ()  [unwired: 2 in, 2 out]
            n169 = property on="Test Slider" class="Slide (strict)"("Visible"=w291) -> ()  [unwired: 2 in, 2 out]
            n170 = Search and Replace String(input string=w292, search string="/Value  **", replace string="/Direction") -> (result string=w298:string)  [unwired: 5 in, 3 out]
            n171 = property on="Test Ring" class="Ring (strict)"("Visible"=w291) -> ()  [unwired: 2 in, 2 out]
            n172 = call <vilib>:"NT Read String.vi"("Name"=w298) -> ("String"=w296:string)  [unwired: 9 in, 1 out]
            n173 = Equal?(x="Both directions", y=w296) -> (x = y?=w294:bool)
            n174 = Not(x=w294) -> (.not. x?=w295:bool)
            n175 = property on="Rev/Fwd" class="Clust (strict)"("Visible"=w294) -> ()  [unwired: 2 in, 2 out]
            n176 = property on="On/Off" class="Bool (strict)"("Visible"=w295, "Caption.Text"=w293) -> ()  [unwired: 2 in, 2 out]
          }
          frame "Compressor", "Digital Out" {
            w301 = FALSE ("Visible")
            # "Get direction and finish"
            n177 = property on="Motor" class="Clust (strict)"("Visible"=w301) -> ()  [unwired: 2 in, 2 out]
            n178 = property on="Test Slider" class="Slide (strict)"("Visible"=w301) -> ()  [unwired: 2 in, 2 out]
            n179 = property on="Test Ring" class="Ring (strict)"("Visible"=w301) -> ()  [unwired: 2 in, 2 out]
            n180 = property on="On/Off" class="Bool (strict)"("Visible"=TRUE, "Caption.Text"=w302) -> ()  [unwired: 2 in, 2 out]
            n181 = property on="Rev/Fwd" class="Clust (strict)"("Visible"=FALSE) -> ()  [unwired: 2 in, 2 out]
          }
          frame "Camera" {
            n182 = call <vilib>:"Get Last Path Segment.vi"("String in"=w309) -> ("String out"=w310:string)  [unwired: 10 in]
            n183 = property on="On/Off" class="Bool (strict)"("Visible"=FALSE) -> ()  [unwired: 2 in, 2 out]
            n184 = property on="Motor" class="Clust (strict)"("Visible"=FALSE) -> ()  [unwired: 2 in, 2 out]
            n185 = property on="Rev/Fwd" class="Clust (strict)"("Visible"=FALSE) -> ()  [unwired: 2 in, 2 out]
            n186 = case shown="\"White Balance  **\"" w310 {
              tunnel: w309 -> [w316 w325 w334 w343 w352 _ w358]
              tunnel: w308 -> [w314 w322 w331 w340 w349 _ _]
              frame "Size  **" {
                n187 = Index Array(array=w314) -> (element=w313:cluster{string[]})  [unwired: 1 in]
                n188 = call <vilib>:"NT Read String.vi"("Name"=w316) -> ("String"=w315:string)  [unwired: 9 in, 1 out]
                n189 = Unbundle(w313) -> (w311:string[])
                n190 = Match First String(2:w311, 3:w315) -> (0:w312:i32)  [unwired: 1 out]
                n191 = property on="Test Ring" class="Ring (strict)"("Value"=w312, "Strings []"=w311) -> ()  [unwired: 2 in, 2 out]
                n192 = property on="Test Ring" class="Ring (strict)"("Visible"=TRUE) -> ()  [unwired: 2 in, 2 out]
                n193 = property on="Test Slider" class="Slide (strict)"("Visible"=FALSE) -> ()  [unwired: 2 in, 2 out]
              }
              frame "White Balance  **" {
                n194 = Index Array(array=w322, index=1) -> (element=w323:cluster{string[]})
                n195 = call <vilib>:"NT Read String.vi"("Name"=w325) -> ("String"=w324:string)  [unwired: 9 in, 1 out]
                n196 = Unbundle(w323) -> (w320:string[])
                n197 = Match First String(2:w320, 3:w324) -> (0:w319:i32)  [unwired: 1 out]
                n198 = property on="Test Ring" class="Ring (strict)"("Value"=w319, "Strings []"=w320) -> ()  [unwired: 2 in, 2 out]
                n199 = property on="Test Ring" class="Ring (strict)"("Visible"=TRUE) -> ()  [unwired: 2 in, 2 out]
                n200 = property on="Test Slider" class="Slide (strict)"("Visible"=FALSE) -> ()  [unwired: 2 in, 2 out]
              }
              frame "Exposure  **" {
                n201 = Index Array(array=w331, index=2) -> (element=w332:cluster{string[]})
                n202 = call <vilib>:"NT Read String.vi"("Name"=w334) -> ("String"=w333:string)  [unwired: 9 in, 1 out]
                n203 = Unbundle(w332) -> (w328:string[])
                n204 = Match First String(2:w328, 3:w333) -> (0:w329:i32)  [unwired: 1 out]
                n205 = property on="Test Ring" class="Ring (strict)"("Value"=w329, "Strings []"=w328) -> ()  [unwired: 2 in, 2 out]
                n206 = property on="Test Ring" class="Ring (strict)"("Visible"=TRUE) -> ()  [unwired: 2 in, 2 out]
                n207 = property on="Test Slider" class="Slide (strict)"("Visible"=FALSE) -> ()  [unwired: 2 in, 2 out]
              }
              frame "Exposure Priority  **" {
                n208 = Index Array(array=w340, index=3) -> (element=w341:cluster{string[]})
                n209 = call <vilib>:"NT Read String.vi"("Name"=w343) -> ("String"=w342:string)  [unwired: 9 in, 1 out]
                n210 = Unbundle(w341) -> (w337:string[])
                n211 = Match First String(2:w337, 3:w342) -> (0:w338:i32)  [unwired: 1 out]
                n212 = property on="Test Ring" class="Ring (strict)"("Value"=w338, "Strings []"=w337) -> ()  [unwired: 2 in, 2 out]
                n213 = property on="Test Ring" class="Ring (strict)"("Visible"=TRUE) -> ()  [unwired: 2 in, 2 out]
                n214 = property on="Test Slider" class="Slide (strict)"("Visible"=FALSE) -> ()  [unwired: 2 in, 2 out]
              }
              frame "Color Enable  **" {
                n215 = Index Array(array=w349, index=4) -> (element=w350:cluster{string[]})
                n216 = call <vilib>:"NT Read String.vi"("Name"=w352) -> ("String"=w351:string)  [unwired: 9 in, 1 out]
                n217 = Unbundle(w350) -> (w346:string[])
                n218 = Match First String(2:w346, 3:w351) -> (0:w347:i32)  [unwired: 1 out]
                n219 = property on="Test Ring" class="Ring (strict)"("Value"=w347, "Strings []"=w346) -> ()  [unwired: 2 in, 2 out]
                n220 = property on="Test Ring" class="Ring (strict)"("Visible"=TRUE) -> ()  [unwired: 2 in, 2 out]
                n221 = property on="Test Slider" class="Slide (strict)"("Visible"=FALSE) -> ()  [unwired: 2 in, 2 out]
              }
              frame Default {
                n222 = property on="Test Ring" class="Ring (strict)"("Visible"=FALSE) -> ()  [unwired: 2 in, 2 out]
                n223 = property on="Test Slider" class="Slide (strict)"("Visible"=FALSE) -> ()  [unwired: 2 in, 2 out]
              }
              frame "Brightness  **", "Color Level  **", "Compression  **", "FPS  **", "Sharpness  **" {
                n224 = call <vilib>:"NT Read Number.vi"("Name"=w358) -> ("Numeric"=w357:dbl)  [unwired: 9 in, 1 out]
                n225 = local write "Test Slider"(w357) -> ()
                n226 = property on="Test Slider" class="Slide (strict)"("Visible"=TRUE, "Scale.Maximum"=100.0 ("Scale.Range:Maximum")) -> ()  [unwired: 2 in, 2 out]
                n227 = property on="Test Ring" class="Ring (strict)"("Visible"=FALSE) -> ()  [unwired: 2 in, 2 out]
              }
            }
          }
        }
        n228 = property on="Progress" class="Clust (strict)"("Visible"=FALSE) -> ()  [unwired: 2 in, 2 out]
      }
      event "Test Name": Mouse Enter {
        # "Populate the ring with the list of tests"
        n229 = event-data() -> ()  [unwired: 1 in, 1 out]
        n230 = call <vilib>:"NT Read String Array.vi"("Name"="/TestMode/TestList") -> ("String Array"=w366:string[])  [unwired: 9 in, 1 out]
        n231 = Build Array (concatenate)("Select the test to run...", w366) -> (w365:string[])
        n232 = property on="Test Name" class="Ring (strict)"("Strings []"=w365) -> ()  [unwired: 2 in, 2 out]
      }
      event "Test Name": Value Change {
        w368 = FALSE ("Visible")
        # "Tell the robot the test name to run"
        n233 = event-data() -> ("NewVal"=w372:u16)  [unwired: 1 in]
        n234 = property on="Test Name" class="Ring (strict)"() -> ("Strings []"=w373:string[])  [unwired: 2 in, 2 out]
        n235 = local write "Progress"(T7 {"Test Progress"=0, "Test Progress Text"=""} ("Progress")) -> ()
        n236 = Index Array(array=w373, index=w372) -> (element=w371:string)
        n237 = call <vilib>:"NT Write String.vi"("String"=w371, "Name"="/TestMode/TestName") -> ()  [unwired: 9 in, 1 out]
        n238 = property on="Progress" class="Clust (strict)"("Visible"=TRUE) -> ()  [unwired: 2 in, 2 out]
        n239 = property on="Motor" class="Clust (strict)"("Visible"=w368) -> ()  [unwired: 2 in, 2 out]
        n240 = property on="Test Slider" class="Slide (strict)"("Visible"=w368) -> ()  [unwired: 2 in, 2 out]
        n241 = property on="On/Off" class="Bool (strict)"("Visible"=w368) -> ()  [unwired: 2 in, 2 out]
        n242 = property on="Rev/Fwd" class="Clust (strict)"("Visible"=w368) -> ()  [unwired: 2 in, 2 out]
        n243 = property on="Test Ring" class="Ring (strict)"("Visible"=w368) -> ()  [unwired: 2 in, 2 out]
      }
      event "Select Auto": Mouse Enter {
        # "Populate the combo box with the list of autonomous options"
        n244 = event-data() -> ()  [unwired: 1 in, 1 out]
        n245 = call <vilib>:"NT Read String Array.vi"("Name"="Auto List") -> ("String Array"=w375:string[])  [unwired: 9 in, 1 out]
        n246 = property on="Select Auto" class="CmbBox"("Strings[]"=w375) -> ()  [unwired: 2 in, 2 out]
      }
      event "Select Auto": Value Change {
        # "User modified the Auto Selection. Write to NT variable so robot knows."
        n247 = event-data() -> ("NewVal"=w378:string)  [unwired: 1 in]
        n248 = call <vilib>:"NT Write String.vi"("String"=w378, "Name"="Auto Selector") -> ()  [unwired: 9 in, 1 out]
      }
      event "Command Selection": Value Change {
        # "Get the params and show in table"
        n249 = event-data() -> ("NewVal"=w384:i32)  [unwired: 1 in]
        n250 = property on="Command Selection" class="MCListbox (strict)"() -> ("ItemNames"=w382:string[][])  [unwired: 2 in, 2 out]
        n251 = call <vilib>:"WPI_DashboardUpdate Command Params.vi"("NewVal"=w384, "Commands"=w382, "Param Tbl"=w383) -> ()  [unwired: 8 in, 1 out]
      }
      event "Execute Command": Value Change {
        # "Started one, Unique ID holds\nresponse"
        n252 = event-data() -> ()  [unwired: 1 in, 1 out]
        n253 = property on="Command Selection" class="MCListbox (strict)"() -> ("ItemNames"=w395:string[][])  [unwired: 2 in, 2 out]
        n254 = Index Array(array=w395, index (row)="Command Selection", index (col)=0) -> (element=w393:string)
        n255 = call <vilib>:"Invoke Commands.vi"("Command Params"="Command Params", "Function Name"=w393) -> ("Params"=w389:u8, "Started"=w388:bool)  [unwired: 7 in, 1 out]
        n256 = Array Subset(array="Command Params", length (row)=w389) -> (w390:string[][])  [unwired: 3 in]
        n257 = Select(t="Executing" ("Cmd Status"), s=w388, f="" ("Cmd Status")) -> (s? t:f=→"Cmd Status":string)
      }
      event "Command Selection": Double Click {
        n258 = event-data() -> ("Row"=w403:i32)  [unwired: 1 in]
        n259 = property on="Command Selection" class="MCListbox (strict)"() -> ("ItemNames"=w406:string[][])  [unwired: 2 in, 2 out]
        n260 = local read "Command Params"() -> (w402:string[][])
        n261 = Index Array(array=w406, index (row)=w403, index (col)=0) -> (element=w404:string)
        n262 = call <vilib>:"Invoke Commands.vi"("Command Params"=w402, "Function Name"=w404) -> ("Params"=w401:u8, "Started"=w396:bool)  [unwired: 7 in, 1 out]
        n263 = Array Subset(array=w402, length (row)=w401) -> (w400:string[][])  [unwired: 3 in]
        n264 = Select(t="Executing" ("Cmd Status"), s=w396, f="" ("Cmd Status")) -> (s? t:f=w397:string)
        n265 = local write "Cmd Status"(w397) -> ()
      }
      event "CheckList": Double Click {
        # "Shift clears all"
        # "Update symbols on the listbox"
        n266 = event-data() -> ("PlatMods.Shift"=w408:bool, "Row"=w410:i32)  [unwired: 1 in]
        n267 = case shown="True" w408 {
          tunnel: w410 -> [w414 _]
          tunnel: 1 -> [w413 _]
          frame False {
            n268 = property on="CheckList" class="LstBox (strict)"() -> ("Item Symbols"=w412:i32[])  [unwired: 2 in, 2 out]
            n269 = Replace Array Subset(array=w412, new element=w413, index=w414) -> (w411:i32[])
            n270 = property on="CheckList" class="LstBox (strict)"("Item Symbols"=w411) -> ()  [unwired: 2 in, 2 out]
          }
          frame True {
            w415 = 0 ("Top Row")
            n271 = property on="CheckList" class="LstBox (strict)"() -> ("Number of Rows"=w417:u32)  [unwired: 2 in, 2 out]
            n272 = Initialize Array(0, w417) -> (w416:i32[])
            n273 = property on="CheckList" class="LstBox (strict)"("Top Row"=w415, "Value"=w415, "Item Symbols"=w416) -> ()  [unwired: 2 in, 2 out]
          }
        }
      }
      event "CheckList": Key Down {
        # "Update symbols on the listbox\nLeft and right keys check and uncheck"
        n274 = event-data() -> ("VKey"=w421:T20)  [unwired: 1 in]
        n275 = case shown="\"Left\", \"Right\"" w421 {
          selector: w421 -> [w426 _]
          tunnel: eventvkey."Left" ("VKey") -> [w424 _]
          frame "Left", "Right" {
            n276 = Equal?(x=w424, y=w426) -> (x = y?=w425:bool)
            n277 = Select(t=0, s=w425, f=1) -> (s? t:f=w427:i32)
            n278 = property on="CheckList" class="LstBox (strict)"() -> ("Item Symbols"=w430:i32[])  [unwired: 2 in, 2 out]
            n279 = Replace Array Subset(array=w430, new element=w427, index="CheckList") -> (w429:i32[])
            n280 = property on="CheckList" class="LstBox (strict)"("Item Symbols"=w429) -> ()  [unwired: 2 in, 2 out]
          }
          frame Default {
          }
        }
      }
      event "Motor.Enable": Value Change {
        # "When the test mode otor enable helper is set, update that\ntree row item's value"
        n281 = event-data() -> ("NewVal"=w436:bool)  [unwired: 1 in]
        n282 = Unbundle("Motor") -> ("Value"=w435:dbl)  [unwired: 1 out]
        n283 = Select(t=w435, s=w436, f=0.0) -> (s? t:f=w433:dbl)
        n284 = call <vilib>:"NT Write Number.vi"("Numeric"=w433, "Name"=w432) -> ()  [unwired: 9 in, 1 out]
      }
      event "Test Slider": Value Change {
        # "When the test mode slider helper is set, update that\ntree row item's value"
        n285 = event-data() -> ("NewVal"=w439:dbl)  [unwired: 1 in]
        n286 = call <vilib>:"NT Write Number.vi"("Numeric"=w439, "Name"=w440) -> ()  [unwired: 9 in, 1 out]
      }
      event "On/Off": Value Change {
        # "When the test mode on/off helper value is set, update that\ntree row item's value"
        n287 = event-data() -> ("NewVal"=w444:bool)  [unwired: 1 in]
        n288 = Boolean To (0,1)(Boolean=w444) -> (0, 1=w443:i16)
        n289 = call <vilib>:"NT Write Number.vi"("Numeric"=w443, "Name"=w442) -> ()  [unwired: 9 in, 1 out]
      }
      event "Rev/Fwd": Value Change {
        # "When the test mode helper value for relays is set, update that\ntree row item's value"
        n290 = event-data() -> ("NewVal.Forward"=w452:bool, "NewVal.Reverse"=w451:bool)  [unwired: 1 in]
        n291 = Boolean To (0,1)(Boolean=w452) -> (0, 1=w448:i16)
        n292 = Boolean To (0,1)(Boolean=w451) -> (0, 1=w450:i16)
        n293 = Negate(x=w450) -> (-x=w449:i16)
        n294 = Add(x=w448, y=w449) -> (x+y=w447:i16)
        n295 = call <vilib>:"NT Write Number.vi"("Numeric"=w447, "Name"=w446) -> ()  [unwired: 9 in, 1 out]
      }
      event "Test Ring": Value Change {
        # "When a test mode helper value is selected from the ring,\nset the tree item's variable to the string value"
        n296 = event-data() -> ("NewVal"=w456:u16)  [unwired: 1 in]
        n297 = property on="Test Ring" class="Ring (strict)"() -> ("Strings []"=w457:string[])  [unwired: 2 in, 2 out]
        n298 = Index Array(array=w457, index=w456) -> (element=w455:string)
        n299 = call <vilib>:"NT Write String.vi"("String"=w455, "Name"=w454) -> ()  [unwired: 9 in, 1 out]
      }
      event "Rec Mode": Value Change {
        # "Update globals for recording mode and path to read log from.\nClear when logging and let NetworkTables set path for vision to\nuse."
        n300 = event-data() -> ("NewVal"=w468:enum32{"Stop", "Record", "Playback"})  [unwired: 1 in]
        n301 = global write "WPI_DashboardLogging Global.vi" "Logging Filename"(path "") -> ()
        n302 = global write "WPI_DashboardLogging Global.vi" "Recording"(w468) -> ()
        n303 = case shown="\"Playback\"" w468 {
          tunnel: w467 -> [_ w470 w479]
          tunnel: [_ _ w478] -> w465
          tunnel: [_ _ w477] -> _
          tunnel: w463 -> [_ _ w475]
          tunnel: cluster{i32, i32} {-250, 170} -> [_ _ w474]
          tunnel: [_ _ T21 {"Image Size"=TRUE, "Image Type"=TRUE, "Pixel Value"=TRUE, "ROI Information"=TRUE, "Zoom Factor"=FALSE} ("Image Information Shown:All Elements")] -> w461
          tunnel: [_ _ TRUE ("Zoom Factor")] -> w460
          tunnel: w459 -> [_ _ w471]
          frame Default {
          }
          frame "Stop", "Record" {
            # "Place Window too"
            n304 = invoke class="VI" method="FP.Close"(reference=w470) -> (reference out=w469:refnum<vi>)  [unwired: 2 in, 2 out]
            n305 = invoke class="VI" method="Abort VI"(reference=w469) -> ()  [unwired: 2 in, 3 out]
          }
          frame "Playback" {
            n306 = call "Open Playback Panel.vi"("Offset"=w474, "DB VI Ref"=w475, "Playback in"=w479) -> ("Playback out"=w476:refnum<vi>)  [unwired: 8 in]
            n307 = register-events(w476, w471) -> (reference out=w478:refnum<event-registration>, error out=w477:errorcluster)  [unwired: 2 in]
          }
        }
        n308 = property on="Camera Image" class="ImageControl"("Image Information Shown"=w461, "Image Information Visible"=w460) -> ()  [unwired: 2 in, 2 out]
        n309 = call <vilib>:"WPI_DashboardNT Log FieldName Cache.vi"("Operation"=enum16{"Lookup/Add", "Index", "Clear"}."Clear") -> ()  [unwired: 8 in, 3 out]
      }
      event Panel Close {
        w481 = enum32{"Stop", "Record", "Playback"}."Stop" ("Rec Mode")
        # "Playback window has been closed, abort"
        n310 = event-data() -> ()  [unwired: 1 in, 4 out]
        n311 = local write "Rec Mode"(w481) -> ()
        n312 = global write "WPI_DashboardLogging Global.vi" "Recording"(w481) -> ()
      }
      event Panel Close {
        # "Abort playback window and ourself"
        n313 = event-data() -> ()  [unwired: 1 in, 4 out]
        n314 = invoke class="VI" method="FP.Close"(reference=w485) -> (reference out=w484:refnum<vi>)  [unwired: 2 in, 2 out]
        n315 = invoke class="VI" method="Abort VI"(reference=w484) -> (error out=w483:errorcluster)  [unwired: 2 in, 2 out]
        n316 = invoke class="VI" method="Abort VI"(error in=w483) -> ()  [unwired: 2 in, 3 out]
      }
      event User Event {
        n317 = event-data() -> ("IDs"=w492:cluster{"RPC field ID":u16, "Unique ID":u16}, "String"=w491:string)  [unwired: 1 in]
        n318 = Bundle("IDs"=w492, "String"=w491) -> (w490:T9)  [unwired: 1 in]
        n319 = call <vilib>:"Retrieve RPC Response.vi"("RPC Response"=w490) -> ("Output"=w488:string[][])  [unwired: 10 in]
        n320 = Build Array (concatenate)(w486, w488) -> (w487:string[][])
        n321 = local write "Command Params"(w487) -> ()
        n322 = local write "Cmd Status"("" ("Cmd Status")) -> ()
      }
      event "Tree": Double Click {
        n323 = event-data() -> ("PlatMods"=w496:T24, "Tag"=w495:string)  [unwired: 1 in]
        n324 = Unbundle(w496) -> ("Shift"=w494:bool)  [unwired: 4 out]
        n325 = Not(x=w494) -> (.not. x?=w493:bool)
        n326 = call <vilib>:"NT Update Persistence.vi"("Persistence"=w493, "Name"=w495) -> ()  [unwired: 9 in, 1 out]
      }
    }
  }
  n327 = while {
    tunnel: w64 -> [w499]
    i -> [w502]
    stop <- FALSE stop-if-true
    n328 = Wait (ms)(milliseconds to wait=u32 100) -> ()  [unwired: 1 out]
    n329 = case shown="\"Playback\"" "Rec Mode" {
      tunnel: w502 -> [_ _ w517]
      tunnel: [u32 2829099 ("Base Color") u32 11141120 ("Target Color") w506] -> w498
      frame "Stop", Default {
        # "Reset the color, extra updates don't cost much"
      }
      frame "Record" {
      }
      frame "Playback" {
        # "Playback"
        n330 = Quotient & Remainder(x=w517, y=u32 50 ("milliseconds to wait")) -> (x-y*floor(x/y)=w513:u32)  [unwired: 1 out]
        n331 = Divide(x=w513, y=u32 50 ("milliseconds to wait")) -> (x/y=w510:dbl)
        n332 = Multiply(x=6.283185307179586, y=w510) -> (x*y=w515:dbl)
        n333 = Sine(x=w515) -> (sin(x)=w514:dbl)
        n334 = Absolute Value(x=w514) -> (abs(x)=w507:dbl)
        n335 = call "Interpolate RGB Color.vi"("Proportion"=w507, "Target Color"=u32 30976, "Base Color"=u32 2829099) -> ("Result Color"=w506:u32)  [unwired: 8 in]
      }
    }
    n336 = property class="Pane"(reference=w499, "PaneColor"=w498) -> ()  [unwired: 1 in, 2 out]
  }
  n337 = local write "Dashboard Tab"(T3."Drive" ("Dashboard Tab")) -> ()
  n338 = property on="On/Off" class="Bool (strict)"("Visible"=w33) -> ()  [unwired: 2 in, 2 out]
  n339 = property on="Motor" class="Clust (strict)"("Visible"=w33) -> ()  [unwired: 2 in, 2 out]
  n340 = property on="Progress" class="Clust (strict)"("Visible"=w33) -> ()  [unwired: 2 in, 2 out]
  n341 = property on="Test Ring" class="Ring (strict)"("Visible"=w33) -> ()  [unwired: 2 in, 2 out]
  n342 = property on="Rev/Fwd" class="Clust (strict)"("Visible"=w33) -> ()  [unwired: 2 in, 2 out]
  n343 = while {
    tunnel: u16 1741 ("timeout ms (25000)") -> [w519]
    stop <- FALSE stop-if-true
    n344 = TCP Create Listener(10:w519) -> (0:w518:errorcluster, 3:w520:refnum<k5>)  [unwired: 4 in, 1 out]
    n345 = case shown="No Error" w518 {
      selector: w518 -> [w522 _]
      tunnel: w520 -> [w523 _]
      frame No Error {
        n346 = while {
          tunnel: w523 -> [w526]
          tunnel: w522 -> [w525]
          stop <- FALSE stop-if-true
          n347 = TCP Wait On Listener(8:w525, 11:w526) -> (0:w527:errorcluster, 4:w528:refnum<k5>)  [unwired: 2 in, 3 out]
          n348 = local write "TCP"(w528) -> ()
          n349 = case shown="No Error" w527 {
            frame No Error {
            }
            frame Error {
              n350 = Wait (ms)(milliseconds to wait=u32 1000) -> ()  [unwired: 1 out]
            }
          }
        }
      }
      frame Error {
        n351 = Wait (ms)(milliseconds to wait=u32 1000) -> ()  [unwired: 1 out]
      }
    }
  }
  n352 = local write "Command Selection"(u16 0 ("milliseconds to wait")) -> ()
  n353 = local write "Command Params"(string[][] [] ("Command Params")) -> ()
  n354 = global write "WPI_DashboardLogging Global.vi" "Recording"(w58) -> ()
  n355 = local write "Rec Mode"(w58) -> ()
  n356 = call <vilib>:"NT Write String.vi"("String"="Select Auto", "Name"="Auto Selector") -> ()  [unwired: 9 in, 1 out]
